vi "Control- StepMotor(SubVI).vi"(7 "Frequency (Hz)":u32=200, 8 "error in (no error)":errorcluster, 9 "LINX Resource in":T1={"IO"=enum."Remote", "Interface"=enum."Serial", "LINX Device Config"={"Interface"=enum."Serial", "COM Port"="COM12", "TCP Configuration"={"IP Address"="", "Port"=0}, "Device Family"=2, "Device ID"=5, "Device Name"="Arduino Nano 328\u0000", "TCP Ref"=refnum, "Channels"={"DI"=[0, 1, 2, 3, 4, 5, 6, 7, 8, 9, 10, 11, 12, 13], "DO"=[0, 1, 2, 3, 4, 5, 6, 7, 8, 9, 10, 11, 12, 13], "AI"=[0, 1, 2, 3, 4, 5, 6, 7], "AO"=[], "PWM"=[3, 5, 6, 9, 10, 11], "QE"=[], "UART"=[0], "I2C 2"=[0], "SPI"=[0], "CAN"=[], "Servo"=[0, 1, 2, 3, 4, 5, 6, 7, 8, 9, 10, 11, 12, 13], "AI Ref (V)"=5.0, "AI Resolution (Bits)"=0, "AO Ref (V)"=0.0, "AO Resolution (Bits)"=0}}}, 10 "DIR pin":u8=3, 11 "Pulse pin":u8=4) -> (0 "error out":errorcluster, 3 "LINX Resource out":T1={"IO"=enum."Remote", "Interface"=enum."Serial", "LINX Device Config"={"Interface"=enum."Serial", "COM Port"="COM12", "TCP Configuration"={"IP Address"="", "Port"=0}, "Device Family"=2, "Device ID"=5, "Device Name"="Arduino Nano 328\u0000", "TCP Ref"=refnum, "Channels"={"DI"=[0, 1, 2, 3, 4, 5, 6, 7, 8, 9, 10, 11, 12, 13], "DO"=[0, 1, 2, 3, 4, 5, 6, 7, 8, 9, 10, 11, 12, 13], "AI"=[0, 1, 2, 3, 4, 5, 6, 7], "AO"=[], "PWM"=[3, 5, 6, 9, 10, 11], "QE"=[], "UART"=[0], "I2C 2"=[0], "SPI"=[0], "CAN"=[], "Servo"=[0, 1, 2, 3, 4, 5, 6, 7, 8, 9, 10, 11, 12, 13], "AI Ref (V)"=5.0, "AI Resolution (Bits)"=0, "AO Ref (V)"=0.0, "AO Resolution (Bits)"=0}}})   [LabVIEW 2015]
uses:
  <vilib>/MakerHub/LINX/Private/Type Defs/LINX Ref.ctl
  <vilib>/MakerHub/LINX/Private/Type Defs/Platform.ctl
  <vilib>/MakerHub/LINX/Private/Type Defs/Interface.ctl
  <vilib>/MakerHub/LINX/Private/Device/Type Defs/LINX Device Config.ctl
  <vilib>/MakerHub/LINX/Private/Device/Type Defs/TCP Config.ctl
  <vilib>/MakerHub/LINX/Private/Device/Type Defs/Channels.ctl
  <vilib>/MakerHub/LINX/Public/Peripherals/Digital/Digital Write 1 Chan.vi
  <vilib>/MakerHub/LINX/Public/Peripherals/Digital/Digital Write N Chans.vi
  <vilib>/MakerHub/LINX/Private/Local IO/LinxDigitalWrite.vi
  <vilib>/MakerHub/LINX/Public/Utilities/Check Channel.vi
  <vilib>/MakerHub/LINX/Private/Utilties/Generate Error.vi
  <vilib>/MakerHub/LINX/LMH-LINX.lvlib
  <vilib>/MakerHub/LINX/Private/Device/Device.lvlib
panel:
  in  "Enable pin":u8=2
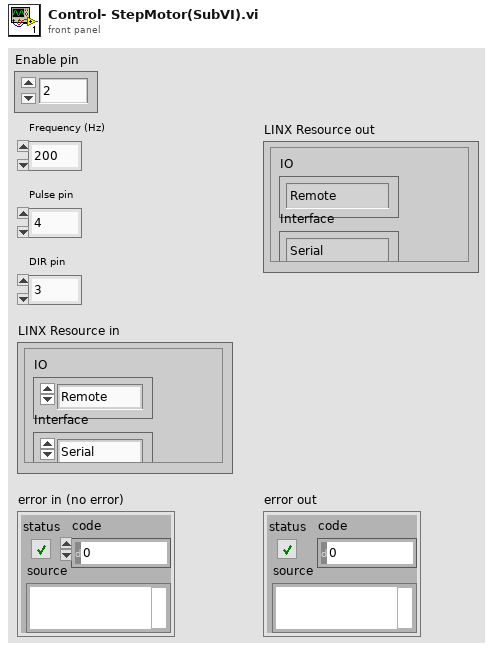
[diagram p1: front panel]
types:
  T1 = typedef "LMH-LINX.lvlib/LINX Ref.ctl" = cluster{"IO":T2, "Interface":T3, "LINX Device Config":T4}
  T2 = typedef "LMH-LINX.lvlib/Platform.ctl" = enum16{"Remote", "Local"}
  T3 = typedef "LMH-LINX.lvlib/Interface.ctl" = enum16{"Serial", "TCP"}
  T4 = typedef "LMH-LINX.lvlib/Device.lvlib/LINX Device Config.ctl" = cluster{"Interface":T3, "COM Port":refnum<visa-resource-name>, "TCP Configuration":T5, "Device Family":u8, "Device ID":u8, "Device Name":string, "TCP Ref":refnum<k5>, "Channels":T6}
  T5 = typedef "LMH-LINX.lvlib/Device.lvlib/TCP Config.ctl" = cluster{"IP Address":string, "Port":u16}
  T6 = typedef "LMH-LINX.lvlib/Channels.ctl" = cluster{"DI":u8[], "DO":u8[], "AI":u8[], "AO":u8[], "PWM":u8[], "QE":u8[], "UART":u8[], "I2C 2":u8[], "SPI":u8[], "CAN":u8[], "Servo":u8[], "AI Ref (V)":dbl, "AI Resolution (Bits)":u8, "AO Ref (V)":dbl, "AO Resolution (Bits)":u8}
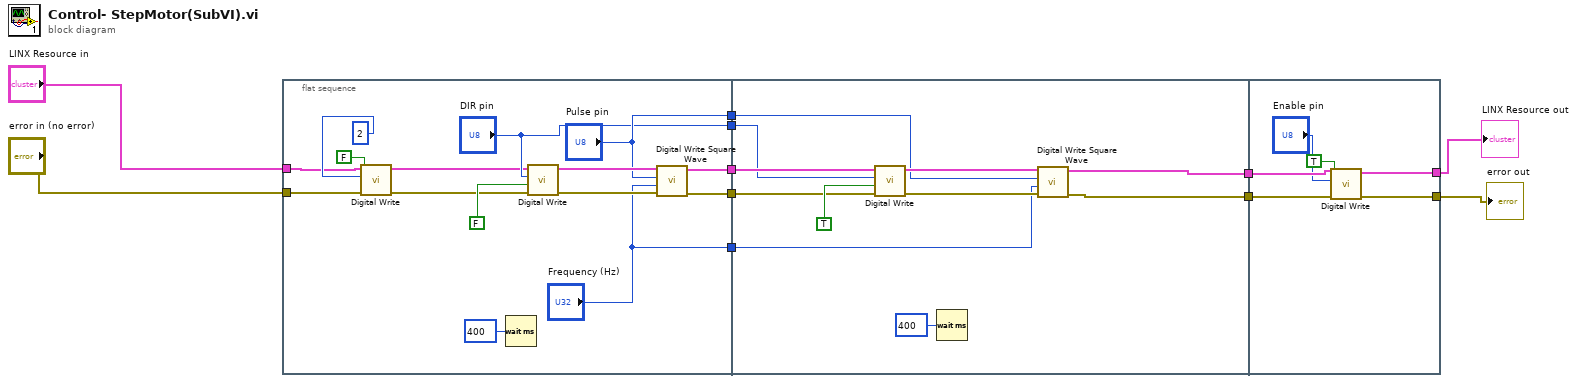
[diagram p0: block diagram]
diagram:
  n1 = flat-sequence {
    tunnel: "LINX Resource in" -> [w15]
    tunnel: "error in (no error)" -> [w14]
    tunnel: [w23] -> w11
    tunnel: [w22] -> w10
    tunnel: ["Frequency (Hz)"] -> w9
    tunnel: ["Pulse pin"] -> w8
    tunnel: ["DIR pin"] -> w7
    tunnel: w11 -> [w34]
    tunnel: w10 -> [w33]
    tunnel: w9 -> [w32]
    tunnel: w8 -> [w31]
    tunnel: w7 -> [w30]
    tunnel: [w28] -> w4
    tunnel: [w27] -> w3
    tunnel: w4 -> [w42]
    tunnel: w3 -> [w41]
    tunnel: [w40] -> w2
    tunnel: [w39] -> w1
    frame #0 {
      n2 = call-poly <vilib>:"Digital Write.vi"("Error In"=w14, "Output Value"=FALSE, "DO Channel"=u8 2, "LINX Resource"=w15) -> ("Error Out"=w12:errorcluster, "LINX Resource"=w13:T1)  [unwired: 6 in]
      n3 = Wait (ms)(milliseconds to wait=u32 400) -> ()  [unwired: 1 out]
      n4 = call-poly <vilib>:"Digital Write.vi"("Error In"=w12, "Output Value"=FALSE, "DO Channel"="DIR pin", "LINX Resource"=w13) -> ("Error Out"=w25:errorcluster, "LINX Resource"=w26:T1)  [unwired: 6 in]
      n5 = call <vilib>:"Digital Write Square Wave.vi"("Error In"=w25, "Frequency (Hz)"="Frequency (Hz)", "Channel"="Pulse pin", "LINX Resource"=w26) -> ("Error Out"=w22:errorcluster, "LINX Resource"=w23:T1)  [unwired: 6 in]
    }
    frame #1 {
      n6 = call-poly <vilib>:"Digital Write.vi"("Error In"=w33, "Output Value"=TRUE, "DO Channel"=w30, "LINX Resource"=w34) -> ("Error Out"=w36:errorcluster, "LINX Resource"=w37:T1)  [unwired: 6 in]
      n7 = Wait (ms)(milliseconds to wait=u32 400) -> ()  [unwired: 1 out]
      n8 = call <vilib>:"Digital Write Square Wave.vi"("Error In"=w36, "Frequency (Hz)"=w32, "Channel"=w31, "LINX Resource"=w37) -> ("Error Out"=w27:errorcluster, "LINX Resource"=w28:T1)  [unwired: 6 in]
    }
    frame #2 {
      n9 = call-poly <vilib>:"Digital Write.vi"("Error In"=w41, "Output Value"=TRUE, "DO Channel"="Enable pin", "LINX Resource"=w42) -> ("Error Out"=w39:errorcluster, "LINX Resource"=w40:T1)  [unwired: 6 in]
    }
  }
  "error out" <- w1
  "LINX Resource out" <- w2
